vi "Assert Almost Equal_Float.vi"(3 "Execution time (s)":dbl=-1.0, 4 "Use Percentage of X (F)":bool, 6 "error code (1)":i32=1, 7 "Label":string, 8 "error in":errorcluster, 9 "Tolerance":ext=0.00000100000000000000000004, 10 "Y":ext, 11 "X":ext) -> (0 "error out":errorcluster, 2 "Properties":refnum<class "Properties.Assert.lvclass">)   [LabVIEW 2021, in "Bananas.lvlib"]
uses:
  Bananas.lvlib
  <vilib>/addons/_JKI Toolkits/Caraya/classes/Assert/Assert.lvclass
  Banana/Banana.lvclass
  AssertTrue/AssertTrue.lvclass
  C:/Repositories/LVOS/Bananas/lv-src/Bananas/AssertTrue/AssertTrue.lvclass
  C:/Repositories/LVOS/Bananas/lv-src/Bananas/BananaPeel/BananaPeel.lvclass
  <vilib>/addons/_JKI Toolkits/Caraya/classes/Properties.Assert/Properties.Assert.lvclass
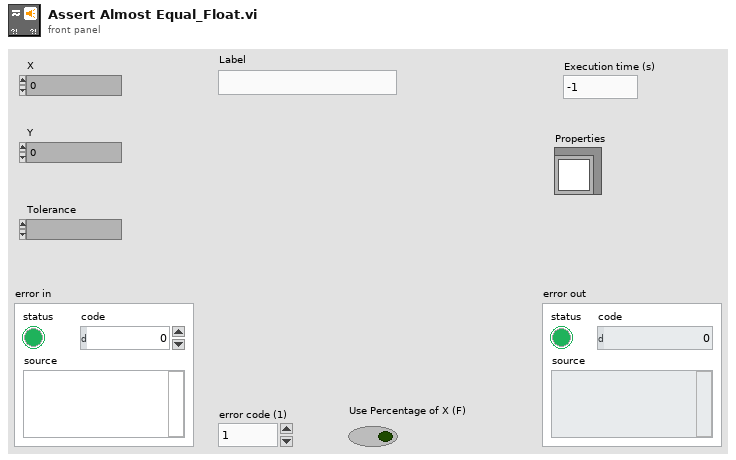
[diagram p1: front panel]
types:
  T1 = typedef "Bananas.lvlib/Assertion Strategies -- cluster.ctl" = cluster{"AssertTrue":refnum<class "AssertTrue.lvclass">, "AssertFalse":refnum<class "AssertFalse.lvclass">}
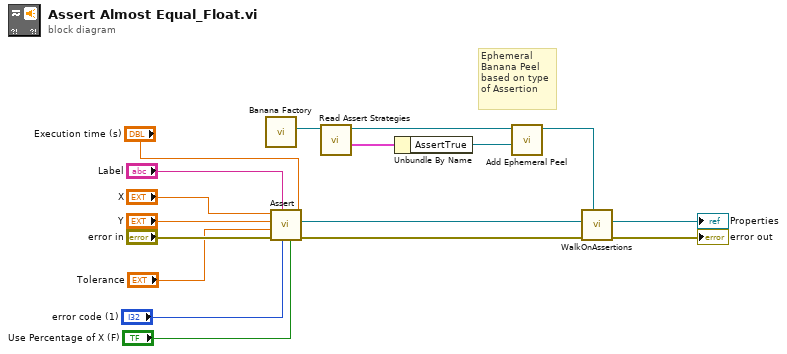
[diagram p0: block diagram]
diagram:
  # "Ephemeral\nBanana Peel\nbased on type\nof Assertion"
  n1 = call "Banana Factory.vi"() -> ("Bunch"=w7:refnum<class "Banana.lvclass">)  [unwired: 10 in, 1 out]
  n2 = call-poly <vilib>:"Assert.vi"("Execution time (s)"="Execution time (s)", "Use Percentage of X (F)"="Use Percentage of X (F)", "error code (1)"="error code (1)", "Label"="Label", "error in (no error)"="error in", "Tolerance"="Tolerance", "Y"="Y", "X"="X") -> ("error out"=w13:errorcluster, "Properties.Assert"=w11:refnum<class "Properties.Assert.lvclass">)  [unwired: 2 in]
  n3 = call "Read Assert Strategies.vi"("Banana in"=w7) -> ("Strategies"=w5:T1, "Banana out"=w6:refnum<class "Banana.lvclass">)  [unwired: 9 in]
  n4 = Unbundle By Name(w5) -> ("AssertTrue"=w8:refnum<class "AssertTrue.lvclass">)
  n5 = call "Add Ephemeral Peel.vi"("BananaPeel"=w8, "Bunch"=w6) -> ("Bunch"=w9:refnum<class "Banana.lvclass">)  [unwired: 9 in]
  n6 = call "WalkOnAssertions.vi"("Bunch"=w9, "error in (no error)"=w13, "Properties"=w11) -> ("error out"=→"error out":errorcluster, "Properties out"=→"Properties":refnum<class "Properties.Assert.lvclass">)  [unwired: 7 in]
